vi "Memory.Globals.vi"() -> ()   [LabVIEW 2016, in "LabVIEW Memory Manager.lvlib"]
uses:
  LabVIEW Memory Manager.lvlib
panel:
  in  "library name":string="LabVIEW Memory Manager.lvlib"
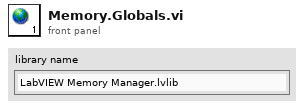
[diagram p1: front panel]
diagram:
